vi "READ_P.vi"(8 "error in (no error)":errorcluster) -> (0 "error out":errorcluster, 3 "value":T1(array[cluster]))   [LabVIEW 2020, in "Productos.lvlib"]
uses:
  Productos.lvlib
  <vilib>/Utility/xml.llb/Read From XML File(string).vi
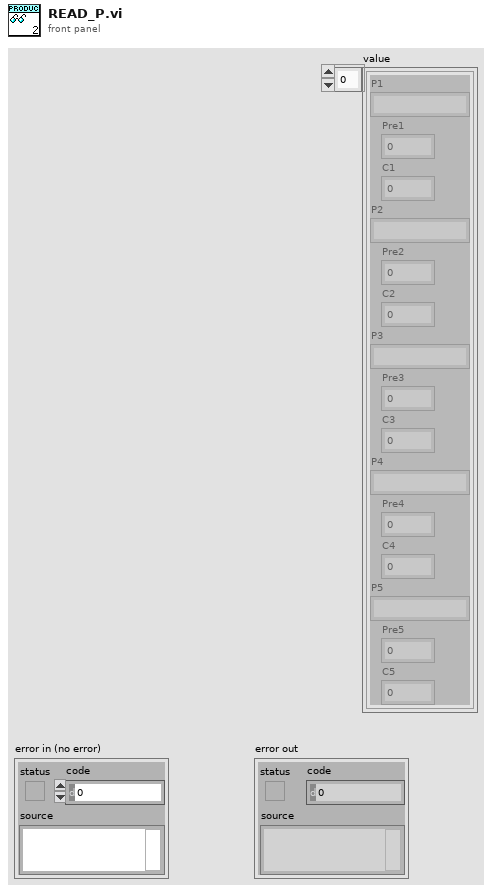
[diagram p1: front panel]
types:
  T1 = cluster{"P1":string, "Pre1":dbl, "C1":dbl, "P2":string, "Pre2":dbl, "C2":dbl, "P3":string, "Pre3":dbl, "C3":dbl, "P4":string, "Pre4":dbl, "C4":dbl, "P5":string, "Pre5":dbl, "C5":dbl}[]
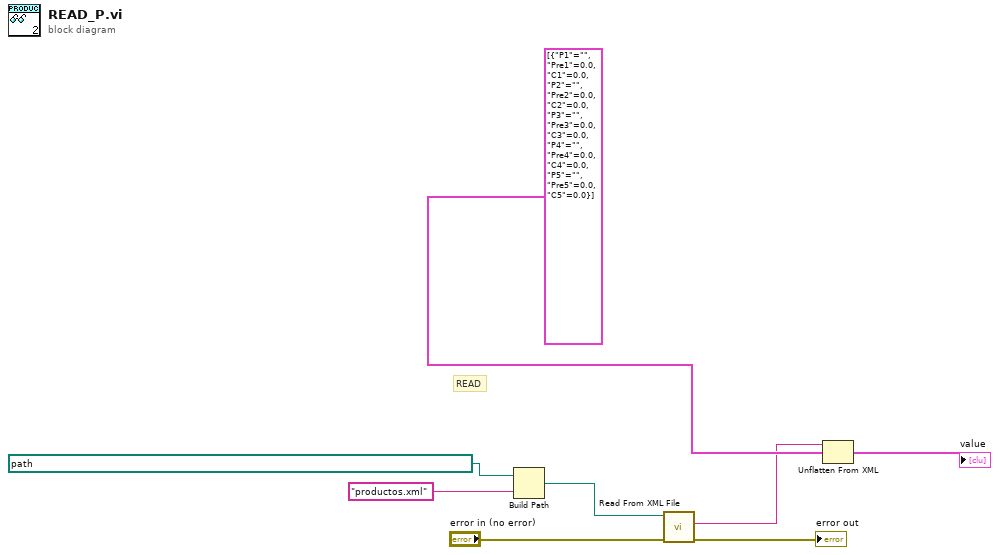
[diagram p0: block diagram]
diagram:
  # "READ"
  n1 = Build Path(base path=path "C:/Users/Ymata/Desktop/séptimo/labview 7mo/Proyecto máuina/Proyecto-maquina", name or relative path="productos.xml") -> (appended path=w6:path)
  n2 = call-poly <vilib>:"Read From XML File.vi"("error in (no error)"="error in (no error)", "XML File Path"=w6) -> ("error out"=→"error out":errorcluster, "XML Elements"=w2:string)  [unwired: 7 in, 1 out]
  n3 = Unflatten From XML(xml string=w2, type=T1 [{"P1"="", "Pre1"=0.0, "C1"=0.0, "P2"="", "Pre2"=0.0, "C2"=0.0, "P3"="", "Pre3"=0.0, "C3"=0.0, "P4"="", "Pre4"=0.0, "C4"=0.0, "P5"="", "Pre5"=0.0, "C5"=0.0}] ("Productos")) -> (value=→"value":T1)  [unwired: 1 in, 1 out]
